vi "BangBang_Calculate_PV.vi"(10 "Measurment":dbl, 11 "BANG_BANG":T1 {"Measurment" format="%13.5p"; "Setpoint" format="%13.5p"; "Tolerance" format="%13.5p"}) -> (1 "ControlOutput":dbl, 3 "out BANG_BANG":T1 {"Measurment" format="%13.5p"; "Setpoint" format="%13.5p"; "Tolerance" format="%13.5p"})   [LabVIEW 2019, in "Trajectory_Library.lvlib"]
doc: "Returns the calculated control output.\n \nAlways ensure that your motor controllers are set to \"coast\" before attempting to control them with a bang-bang controller.\n \nInput:\n - BangBang -- Data cluster\n - measurement -- The most recent measurement of the process variable.\n - setpoint -- The setpoint for the process variable.\n\nOutput\n - outBangBang -- Updated data cluster\n - ControlOutput -- The calculated motor output (0 or 1)."
uses:
  BANG_BANG.ctl
  Trajectory_Library.lvlib
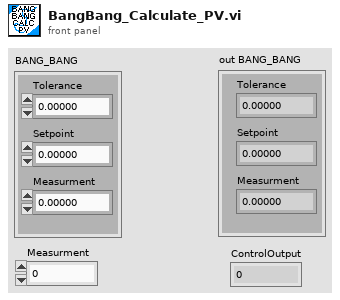
[diagram p1: front panel]
types:
  T1 = typedef "Trajectory_Library.lvlib/BANG_BANG.ctl" = cluster{"Tolerance":dbl, "Setpoint":dbl, "Measurment":dbl}
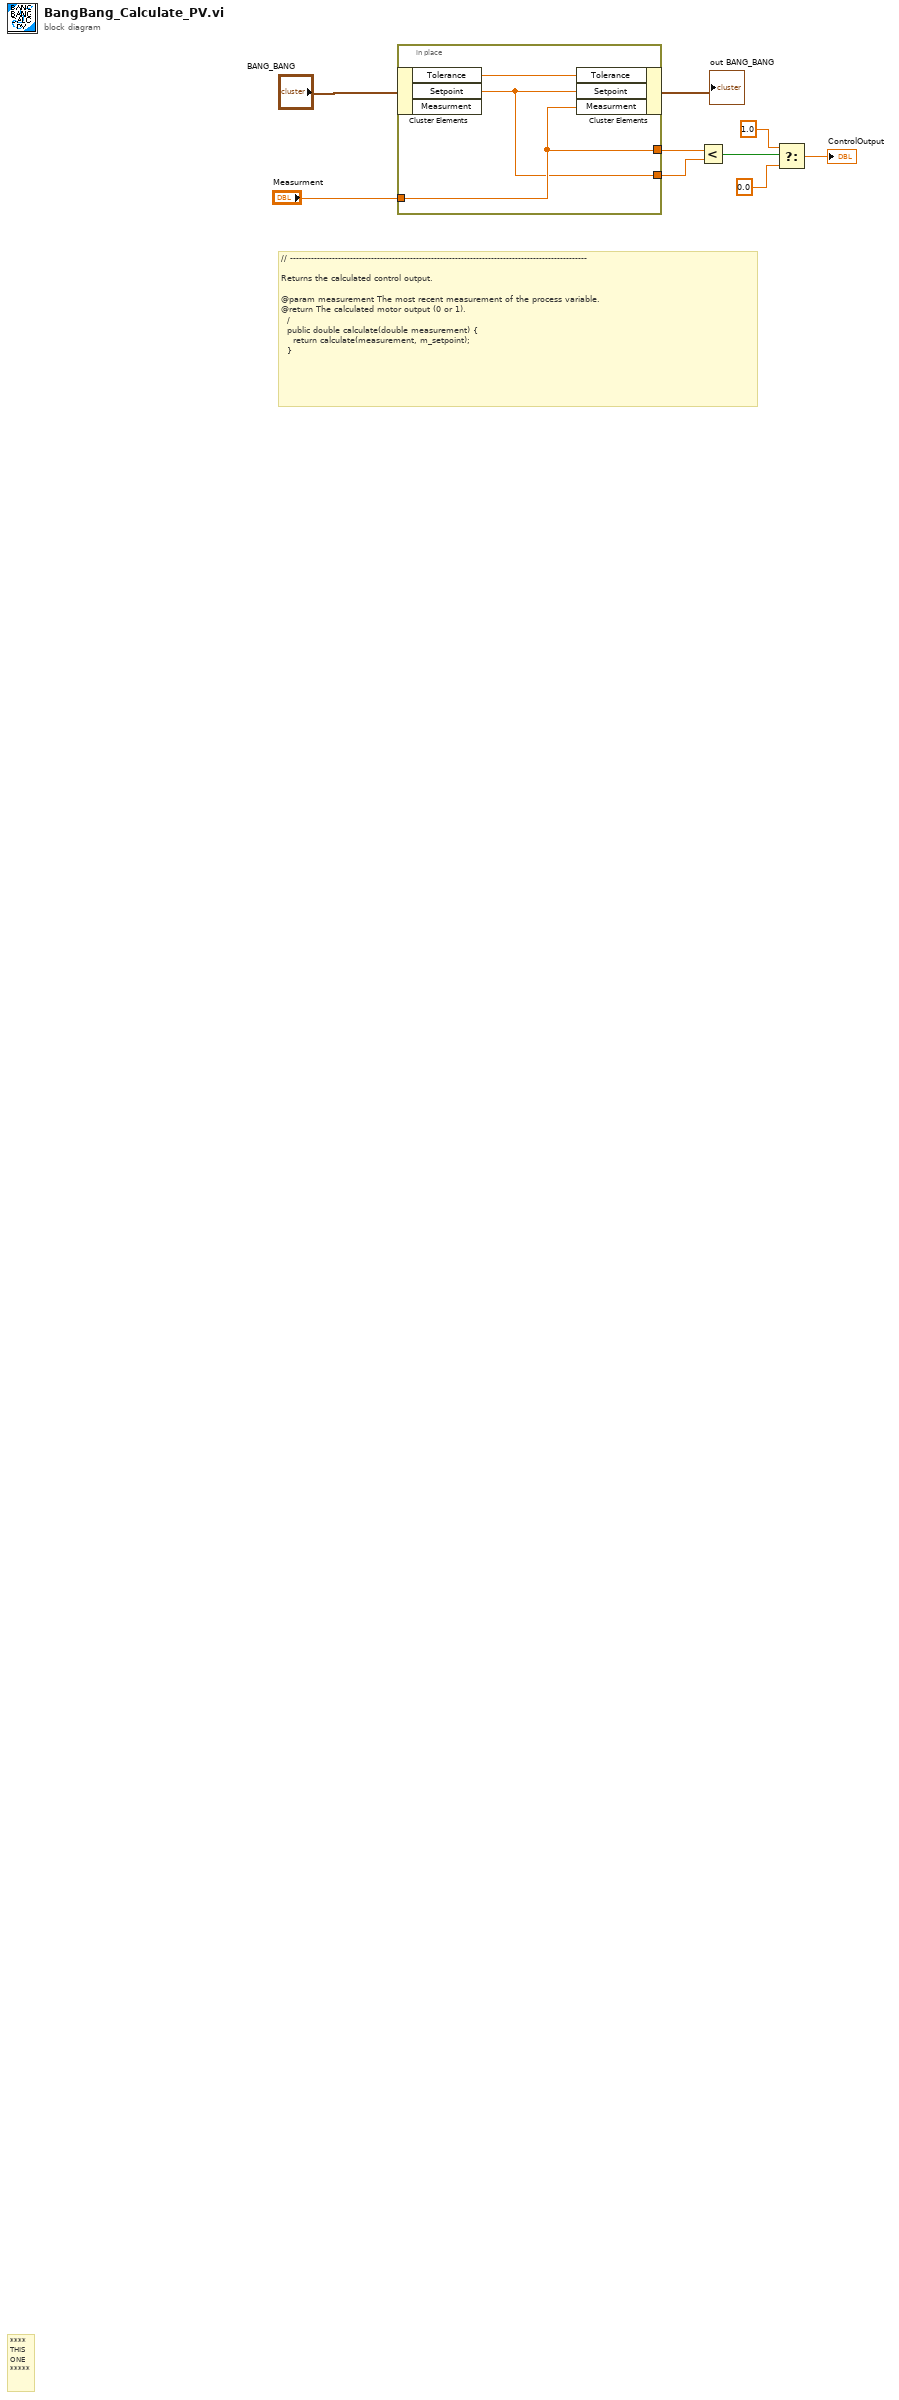
[diagram p0: block diagram]
diagram:
  # "// ---------------------------------------------------------------------------------------------------\n  \nReturns the calculated control output.\n  \n@param measurement The most recent measurement of the process variable.\n@return The calculated motor output (0 or 1).\n  /\n  public double calculate(double measurement) {\n    return calculate(measurement, m_setpoint);\n  }"
  # "****\nTHIS\nONE\n*****"
  n1 = in-place {
    in-place-border: "Measurment" -> [w11]
    in-place-border: [w11] -> w6
    in-place-border: [w10] -> w1
    n2 = in-place-cluster #1("BANG_BANG") -> ("Tolerance"=w12:dbl, "Setpoint"=w10:dbl)  [unwired: 1 out]
    n3 = in-place-cluster #1("Tolerance"=w12, "Setpoint"=w10, "Measurment"=w11) -> (→"out BANG_BANG":T1)
  }
  n4 = Less?(x=w6, y=w1) -> (x < y?=w5:bool)
  n5 = Select(t=1.0, s=w5, f=0.0) -> (s? t:f=→"ControlOutput":dbl)
